vi "LIA7230_channel_percent.vi"(0 "Reference Mode":bool, 1 "Range single mode":u8(ring)=26 items=["N/A", "2nV", "5nV", "10nV", "20nV", "50nV", "100nV", "200nV", "500nV", "1µV", "2µV", "5µV", "10µV", "20µV", "50µV", "100µV", "200µV", "500µV", "1mV", "2mV", "5mV", "10mV", "20mV", "50mV", "100mV", "200mV", "500mV", "1V"], 2 "Display Type":u16(ring)=23 items=["X1 %", "Y1 %", "X1 Calibrated", "Y1 Calibrated", "Mag1 %", "Mag1 Calibrated", "Phase1 Degrees", "Ratio", "Log Ratio", "ADC 1", "ADC 2", "ADC 3", "ADC 4", "Noise1 %", "Noise1 Calibrated", "Ref Frequency 1", "Equation 1", "Equation 2", "X2 %", "Y2 %", "X2 Calibrated", "Y2 Calibrated", "Mag2 %", "Mag2 Calibrated", "Phase2 Degrees"], 3 "Input Mode":u16(ring)=1 items=["Inputs Grounded (test)", "A (Single-Ended Voltage)", "-B (Inverting Single Ended Voltage)", "A-B (Differential Voltage)", "AUX Input - Main Console", "B Current input - Wide Bandwidth", "B Current input - Low Noise"], 4 "Range dual mode":u8(ring)=25 items=["N/A", "2nV", "5nV", "10nV", "20nV", "50nV", "100nV", "200nV", "500nV", "1µV", "2µV", "5µV", "10µV", "20µV", "50µV", "100µV", "200µV", "500µV", "1mV", "2mV", "5mV", "10mV", "20mV", "50mV", "100mV", "200mV", "500mV", "1V"], 5 "Channel signal":dbl) -> (6 "Channel signal percent":dbl, 8 "Channel signal in full range":dbl)   [LabVIEW 2019]
panel:
  # "Dual"
  # "Single"
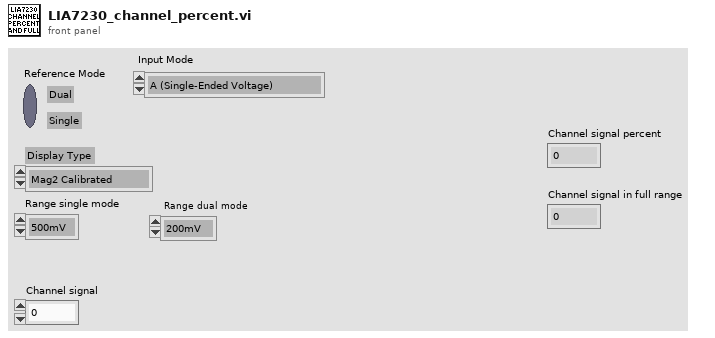
[diagram p1: front panel]
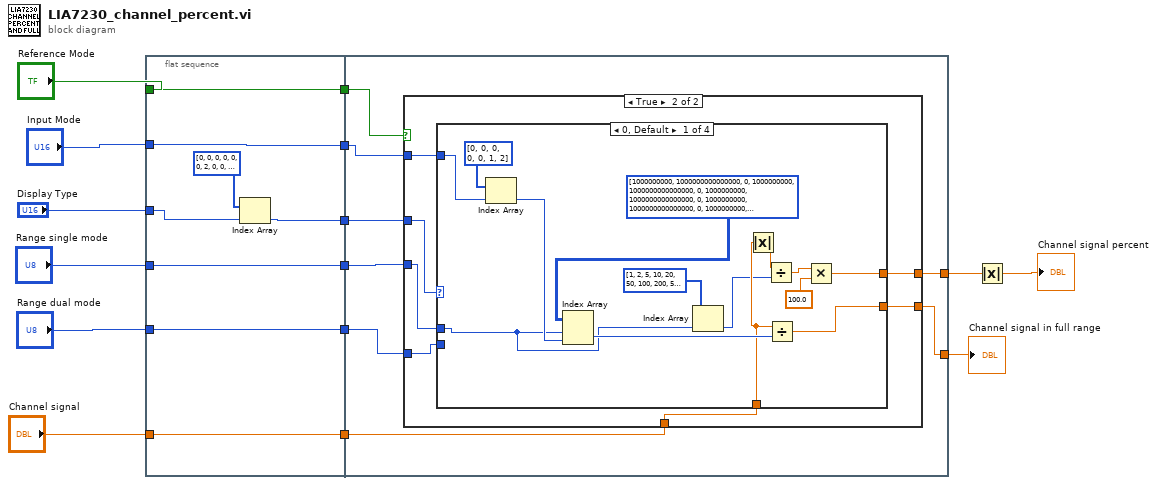
[diagram p0: block diagram]
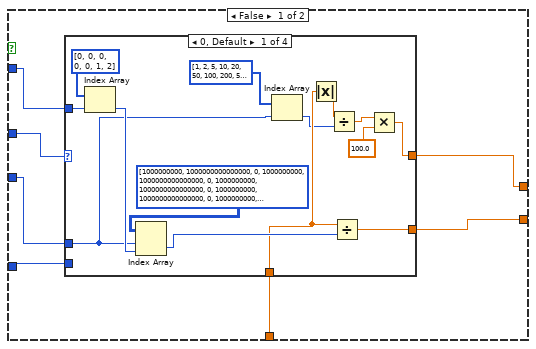
[diagram p2: hidden frame]
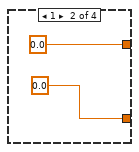
[diagram p3: hidden frame]
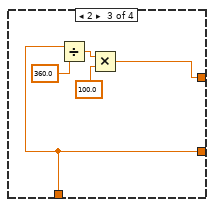
[diagram p4: hidden frame]
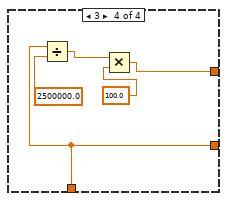
[diagram p5: hidden frame]
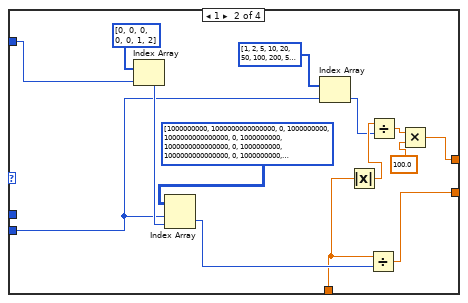
[diagram p6: hidden frame]
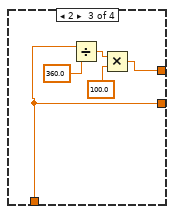
[diagram p7: hidden frame]
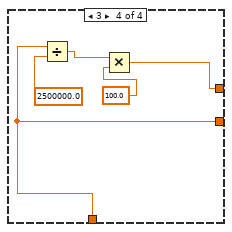
[diagram p8: hidden frame]
diagram:
  n1 = flat-sequence {
    tunnel: "Display Type" -> [w22]
    tunnel: [w21] -> w14
    tunnel: "Reference Mode" -> [w21]
    tunnel: "Input Mode" -> [w20]
    tunnel: [w20] -> w11
    tunnel: [w19] -> w10
    tunnel: "Range single mode" -> [w19]
    tunnel: [w18] -> w8
    tunnel: "Range dual mode" -> [w18]
    tunnel: [w17] -> w6
    tunnel: "Channel signal" -> [w17]
    tunnel: [w16] -> w4
    tunnel: w14 -> [w31]
    tunnel: w11 -> [w28]
    tunnel: w10 -> [w30]
    tunnel: w8 -> [w29]
    tunnel: w6 -> [w26]
    tunnel: w4 -> [w27]
    tunnel: [w25] -> w3
    tunnel: [w24] -> w2
    frame #0 {
      n2 = Index Array(array=i32[] [0, 0, 0, 0, 0, 0, 2, 0, 0, 0, 0, 0, 0, 0, 0, 3, 0, 0, 1, 1, 1, 1, 1, 1, 2], index=w22) -> (element=w16:i32)
    }
    frame #1 {
      n3 = case shown="True" w31 {
        tunnel: w30 -> [w37 w69]
        tunnel: w29 -> [w35 w66]
        tunnel: w28 -> [w38 w70]
        tunnel: w27 -> [w36 w71]
        tunnel: w26 -> [w33 w67]
        tunnel: [w34 w68] -> w25
        tunnel: [w32 w65] -> w24
        frame False {
          n4 = case shown="0, Default" w36 {
            tunnel: w38 -> [w49 _ _ _]
            tunnel: w37 -> [w45 _ _ _]
            tunnel: w35 -> [_ _ _ _]
            tunnel: [w48 0.0 w55 w60] -> w34
            tunnel: w33 -> [w41 _ w55 w60]
            tunnel: [w39 0.0 w56 w61] -> w32
            frame 0, Default {
              n5 = Index Array(array=i32[] [0, 0, 0, 0, 0, 1, 2], index=w49) -> (element=w50:i32)
              n6 = Index Array(array=u64[][] [[1000000000, 1000000000000000, 0], [1000000000, 1000000000000000, 0], [1000000000, 1000000000000000, 0], [1000000000, 1000000000000000, 0], [1000000000, 1000000000000000, 0], [1000000000, 1000000000000000, 0], [1000000000, 1000000000000000, 0], [1000000000, 1000000000000000, 1000000000000000], [1000000000, 1000000000000000, 1000000000000000], [1000000, 1000000000000, 1000000000000000], [1000000, 1000000000000, 1000000000000000], [1000000, 1000000000000, 1000000000000000], [1000000, 1000000000000, 1000000000000000], [1000000, 1000000000000, 1000000000000000], [1000000, 1000000000000, 1000000000000000], [1000000, 1000000000000, 1000000000000], [1000000, 1000000000000, 1000000000000], [1000000, 1000000000000, 1000000000000], [1000, 1000000000, 1000000000000], [1000, 1000000000, 1000000000000], [1000, 1000000000, 1000000000000], [1000, 1000000000, 1000000000000], [1000, 1000000000, 1000000000000], [1000, 1000000000, 1000000000000], [1000, 1000000000, 1000000000], [1000, 1000000000, 1000000000], [1000, 1000000000, 1000000000], [1, 1000000, 1000000000]], index (row)=w45, index (col)=w50) -> (element=w47:u64)
              n7 = Index Array(array=i32[] [1, 2, 5, 10, 20, 50, 100, 200, 500, 1, 2, 5, 10, 20, 50, 100, 200, 500, 1, 2, 5, 10, 20, 50, 100, 200, 500, 1], index=w45) -> (element=w40:i32)
              n8 = Absolute Value(x=w41) -> (abs(x)=w44:dbl)
              n9 = Divide(x=w44, y=w40) -> (x/y=w43:dbl)
              n10 = Divide(x=w41, y=w47) -> (x/y=w48:dbl)
              n11 = Multiply(x=w43, y=100.0) -> (x*y=w39:dbl)
            }
            frame 1 {
            }
            frame 2 {
              n12 = Divide(x=w55, y=360.0) -> (x/y=w58:dbl)
              n13 = Multiply(x=w58, y=100.0) -> (x*y=w56:dbl)
            }
            frame 3 {
              n14 = Divide(x=w60, y=2500000.0) -> (x/y=w63:dbl)
              n15 = Multiply(x=w63, y=100.0) -> (x*y=w61:dbl)
            }
          }
        }
        frame True {
          n16 = case shown="0, Default" w71 {
            tunnel: w70 -> [w83 w96 _ _]
            tunnel: w69 -> [w77 _ _ _]
            tunnel: [w81 w94 w104 w109] -> w68
            tunnel: w67 -> [w79 w91 w104 w109]
            tunnel: w66 -> [_ w92 _ _]
            tunnel: [w72 w86 w101 w105] -> w65
            frame 0, Default {
              n17 = Index Array(array=i32[] [0, 0, 0, 0, 0, 1, 2], index=w83) -> (element=w84:i32)
              n18 = Index Array(array=u64[][] [[1000000000, 1000000000000000, 0], [1000000000, 1000000000000000, 0], [1000000000, 1000000000000000, 0], [1000000000, 1000000000000000, 0], [1000000000, 1000000000000000, 0], [1000000000, 1000000000000000, 0], [1000000000, 1000000000000000, 0], [1000000000, 1000000000000000, 1000000000000000], [1000000000, 1000000000000000, 1000000000000000], [1000000, 1000000000000, 1000000000000000], [1000000, 1000000000000, 1000000000000000], [1000000, 1000000000000, 1000000000000000], [1000000, 1000000000000, 1000000000000000], [1000000, 1000000000000, 1000000000000000], [1000000, 1000000000000, 1000000000000000], [1000000, 1000000000000, 1000000000000], [1000000, 1000000000000, 1000000000000], [1000000, 1000000000000, 1000000000000], [1000, 1000000000, 1000000000000], [1000, 1000000000, 1000000000000], [1000, 1000000000, 1000000000000], [1000, 1000000000, 1000000000000], [1000, 1000000000, 1000000000000], [1000, 1000000000, 1000000000000], [1000, 1000000000, 1000000000], [1000, 1000000000, 1000000000], [1000, 1000000000, 1000000000], [1, 1000000, 1000000000]], index (row)=w77, index (col)=w84) -> (element=w80:u64)
              n19 = Index Array(array=i32[] [1, 2, 5, 10, 20, 50, 100, 200, 500, 1, 2, 5, 10, 20, 50, 100, 200, 500, 1, 2, 5, 10, 20, 50, 100, 200, 500, 1], index=w77) -> (element=w76:i32)
              n20 = Absolute Value(x=w79) -> (abs(x)=w75:dbl)
              n21 = Divide(x=w75, y=w76) -> (x/y=w74:dbl)
              n22 = Divide(x=w79, y=w80) -> (x/y=w81:dbl)
              n23 = Multiply(x=w74, y=100.0) -> (x*y=w72:dbl)
            }
            frame 1 {
              n24 = Index Array(array=i32[] [0, 0, 0, 0, 0, 1, 2], index=w96) -> (element=w98:i32)
              n25 = Index Array(array=u64[][] [[1000000000, 1000000000000000, 0], [1000000000, 1000000000000000, 0], [1000000000, 1000000000000000, 0], [1000000000, 1000000000000000, 0], [1000000000, 1000000000000000, 0], [1000000000, 1000000000000000, 0], [1000000000, 1000000000000000, 0], [1000000000, 1000000000000000, 1000000000000000], [1000000000, 1000000000000000, 1000000000000000], [1000000, 1000000000000, 1000000000000000], [1000000, 1000000000000, 1000000000000000], [1000000, 1000000000000, 1000000000000000], [1000000, 1000000000000, 1000000000000000], [1000000, 1000000000000, 1000000000000000], [1000000, 1000000000000, 1000000000000000], [1000000, 1000000000000, 1000000000000], [1000000, 1000000000000, 1000000000000], [1000000, 1000000000000, 1000000000000], [1000, 1000000000, 1000000000000], [1000, 1000000000, 1000000000000], [1000, 1000000000, 1000000000000], [1000, 1000000000, 1000000000000], [1000, 1000000000, 1000000000000], [1000, 1000000000, 1000000000000], [1000, 1000000000, 1000000000], [1000, 1000000000, 1000000000], [1000, 1000000000, 1000000000], [1, 1000000, 1000000000]], index (row)=w92, index (col)=w98) -> (element=w95:u64)
              n26 = Index Array(array=i32[] [1, 2, 5, 10, 20, 50, 100, 200, 500, 1, 2, 5, 10, 20, 50, 100, 200, 500, 1, 2, 5, 10, 20, 50, 100, 200, 500, 1], index=w92) -> (element=w89:i32)
              n27 = Absolute Value(x=w91) -> (abs(x)=w90:dbl)
              n28 = Divide(x=w91, y=w95) -> (x/y=w94:dbl)
              n29 = Divide(x=w90, y=w89) -> (x/y=w88:dbl)
              n30 = Multiply(x=w88, y=100.0) -> (x*y=w86:dbl)
            }
            frame 2 {
              n31 = Divide(x=w104, y=360.0) -> (x/y=w102:dbl)
              n32 = Multiply(x=w102, y=100.0) -> (x*y=w101:dbl)
            }
            frame 3 {
              n33 = Divide(x=w109, y=2500000.0) -> (x/y=w107:dbl)
              n34 = Multiply(x=w107, y=100.0) -> (x*y=w105:dbl)
            }
          }
        }
      }
    }
  }
  n35 = Absolute Value(x=w2) -> (abs(x)=→"Channel signal percent":dbl)
  "Channel signal in full range" <- w3
